vi "MainCodeSimple.vi"() -> ()   [LabVIEW 2023]
uses:
  <extravilib>/ChannelInstances/Tag-bool/Read With Abort.vi
  <extravilib>/ChannelInstances/Tag-bool/Write With Abort.vi
  <vilib>/Instr/_visa.llb/VISA Configure Serial Port (Instr).vi
  <extravilib>/ChannelInstances/Tag-bool/Instantiate.vi
  <extravilib>/ChannelInstances/Tag-bool/EndpointRead.vi
  <vilib>/Utility/file.llb/Write Delimited Spreadsheet (DBL).vi
  <extravilib>/ChannelInstances/Tag-bool/Endpoint.vi
  <extravilib>/ChannelInstances/Tag-bool.lvlib
panel:
  in  "Target temp":dbl format="%#_13g"
  in  "Massflow in, see table for ref (mV)":dbl
  in  "Opening, ouptut down (adsorption) (deg)":dbl
  in  "Opening, ouptut up (desorption) (deg)":dbl
  in  "Opening, input (deg)":dbl
  out "Temp PID":dbl(slide) scale=0.0..100.0
  in  "VISA PID":refnum<visa-resource-name>="COM6"
  out "Mode ON/OFF":bool
  out "Mode PID":bool
  in  "Switch Mode":bool
  in  "DC Pulse (ON/OFF)":bool
  in  "Sampling time (ms)":dbl format="%#_13g"
  out "Thermometer 1":dbl(slide) scale=0.0..100.0
  in  "Path":path
  in  "Save data":bool
  in  "Input massflow":dbl format="%#_13g"
  in  "C_CO2":dbl format="%#_13g"
  in  "Temp_e_3":dbl format="%#_13g"
  in  "Temp_e_2":dbl format="%#_13g"
  in  "Temp_e_1":dbl format="%#_13g"
  in  "Temp_m_3":dbl format="%#_13g"
  in  "Temp_m_2":dbl format="%#_13g"
  in  "Temp_m_1":dbl format="%#_13g"
  in  "DAC_2_1":dbl format="%#_13g"
  in  "DAC_2_0":dbl format="%#_13g"
  in  "DAC_1_1":dbl format="%#_13g"
  in  "DAC_1_0":dbl format="%#_13g"
  out "Thermometer 2":dbl(slide) scale=0.0..100.0
  out "error out 3":errorcluster
  in  "VISA Arduino":refnum<visa-resource-name>
  in  "STOP PROGRAM":bool
  # "CONTROL PANEL"
  # "Process"
  # "Serial"
  # "For the moment, mass flows under 100m^3/h are not supported"
  # "For adsorption (90°) and desorption (20°):\n-Adsorption -> 1000mV 208m^3/h\n                            1500mV 307m^3/h\n                            2000mV 406m^3/h\n                            2500mV 505m^3/h\n                            3000mV 604m^3/h\n-Desorption -> 3000mV 200m^3/h \n                           2500mV 180m^3/h \n                           2000mV 130m^3/h \n                           1500mV 100m^3/h"
  # "Careful that PID arduino are not communicating on same port"
  # "MONITORING"
  # "Data save"
  # "CURRENT ACTUATOR VALUES"
  # "PID temperature monitoring"
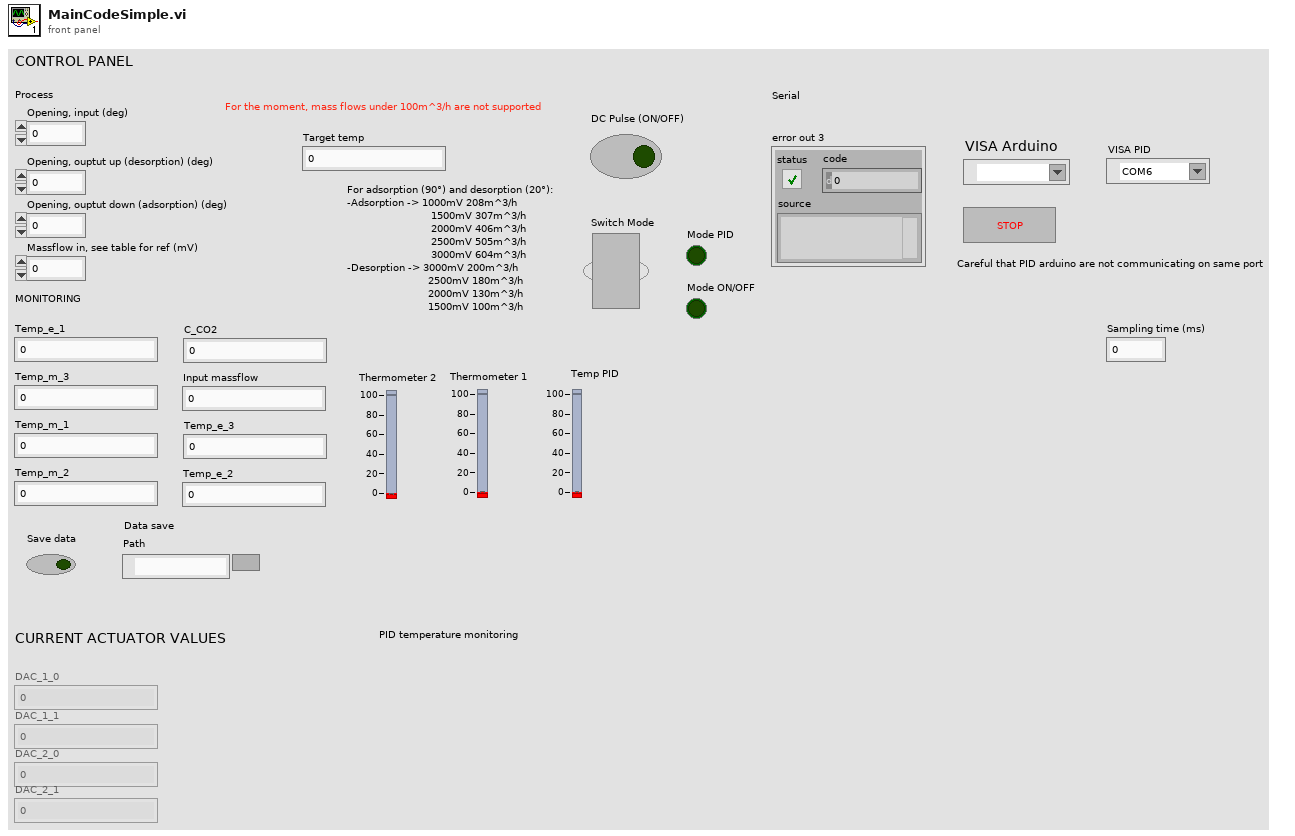
[diagram p1: front panel]
types:
  T1 = typedef "Tag-bool.lvlib/))Channel.ctl" = refnum<queue>
  T2 = cluster{"Temp_m_1":dbl, "Temp_m_2":dbl, "Temp_m_3":dbl, "Temp_e_1":dbl, "Temp_e_2":dbl, "Temp_e_3":dbl, "C_CO2":dbl, "Input massflow":dbl}
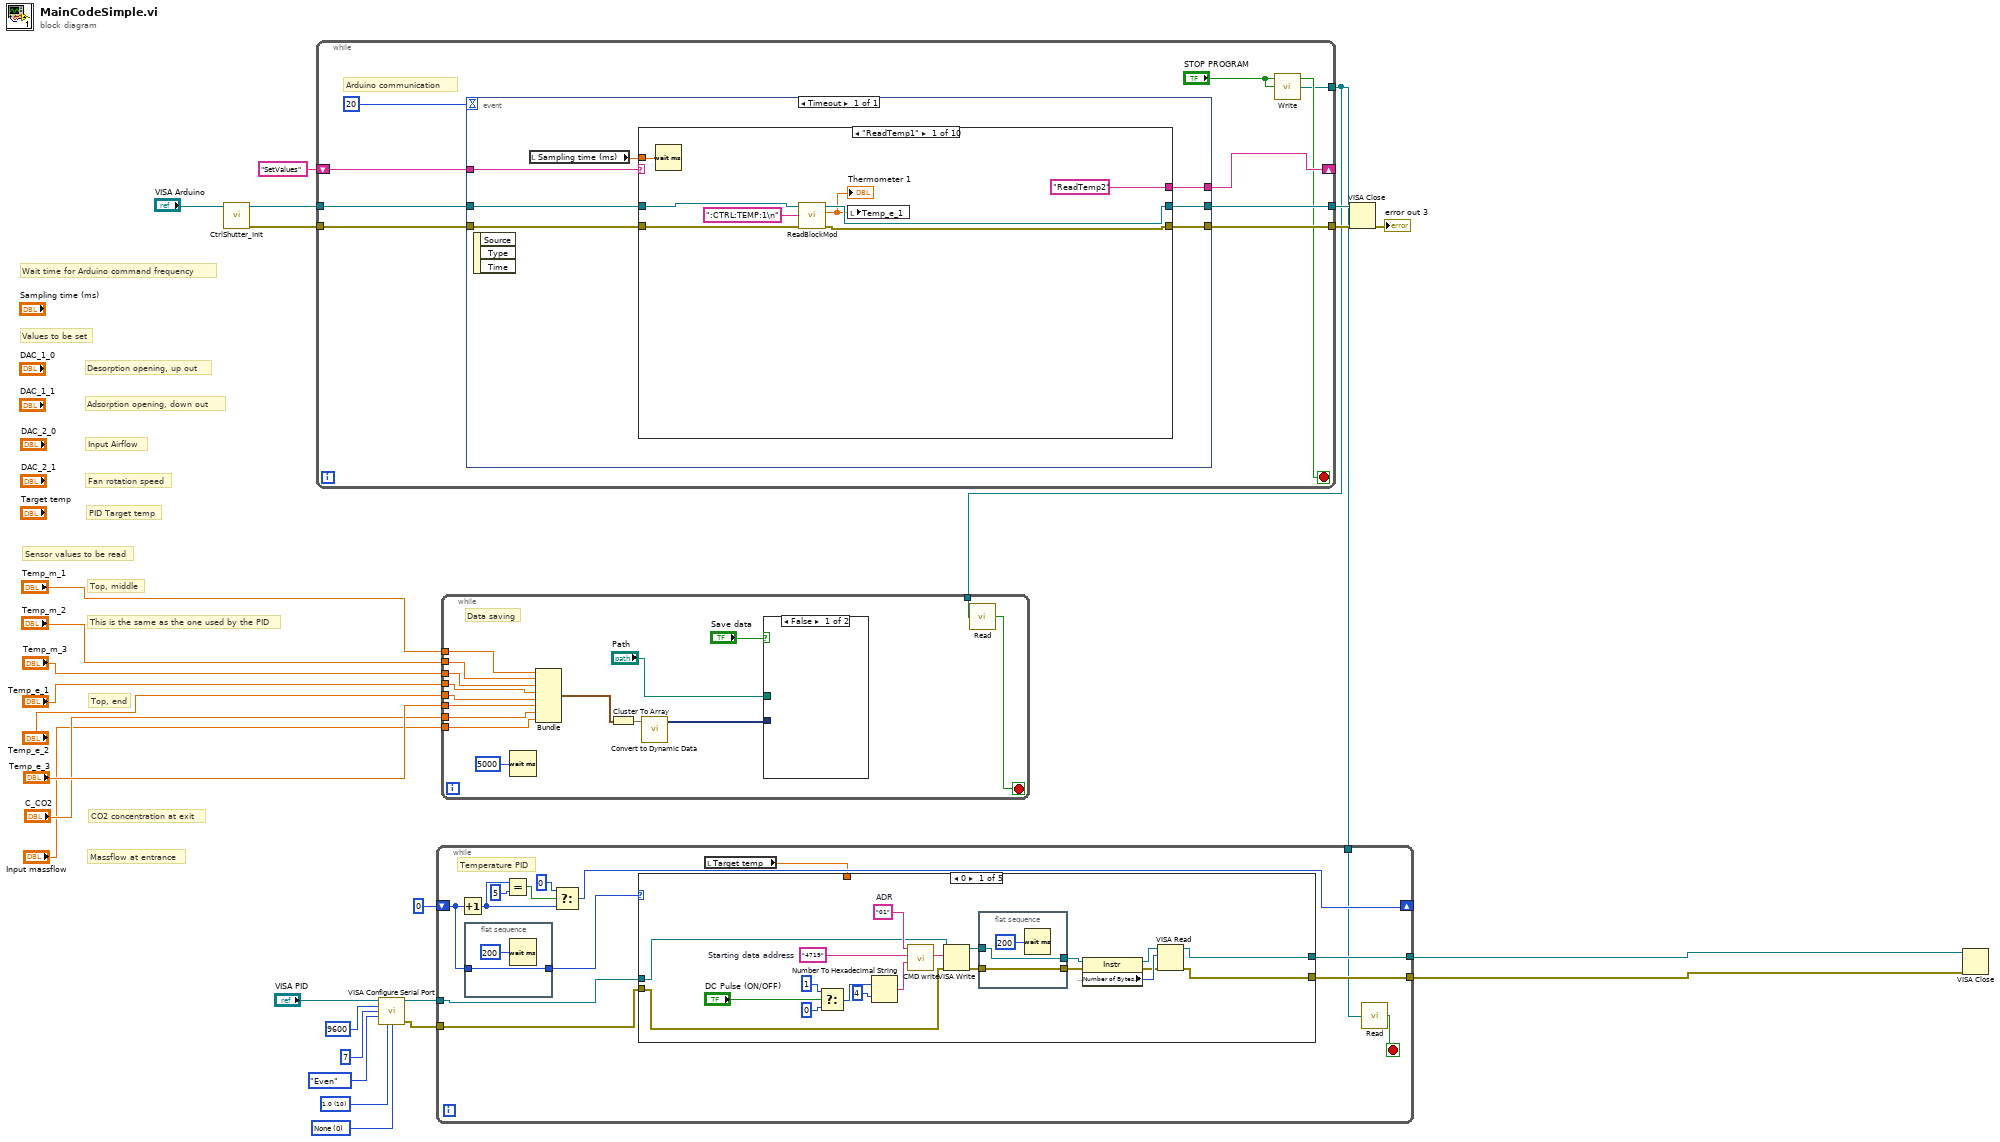
[diagram p0: block diagram]
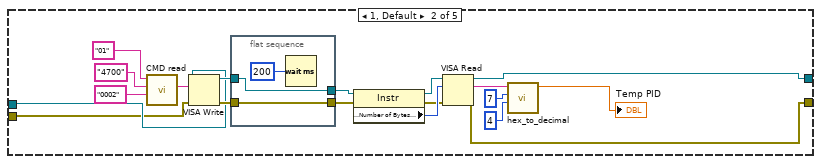
[diagram p2: hidden frame]
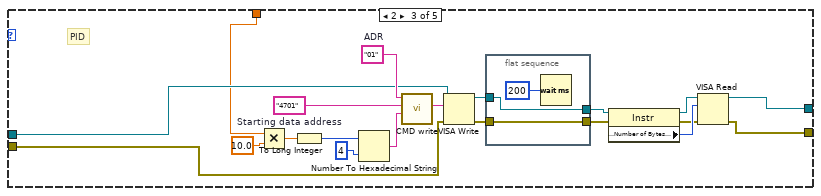
[diagram p3: hidden frame]
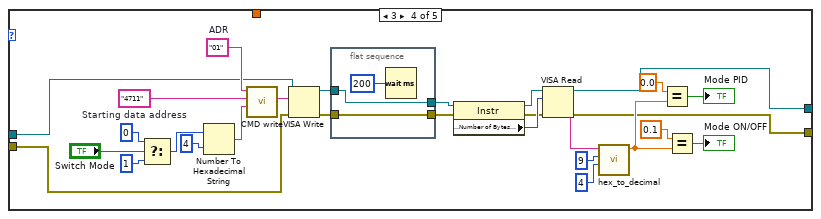
[diagram p4: hidden frame]
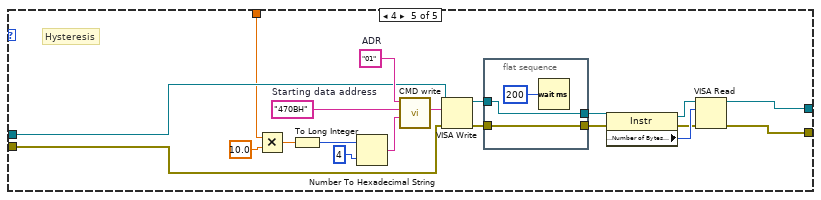
[diagram p5: hidden frame]
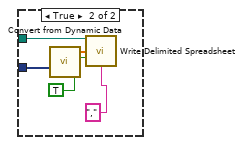
[diagram p6: hidden frame]
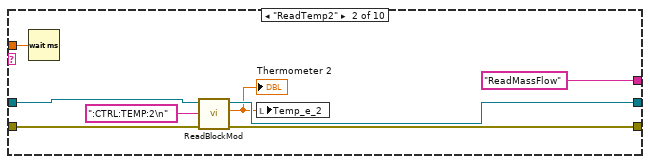
[diagram p7: hidden frame]
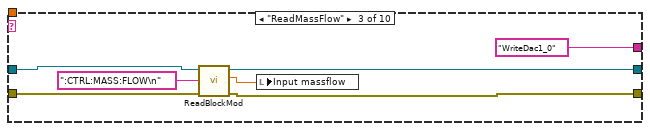
[diagram p8: hidden frame]
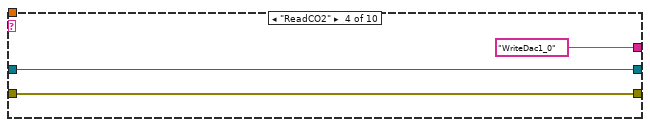
[diagram p9: hidden frame]
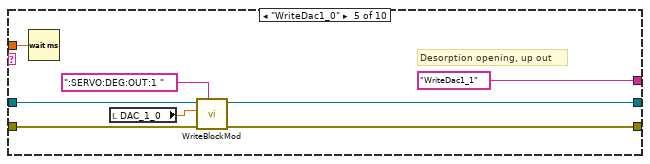
[diagram p10: hidden frame]
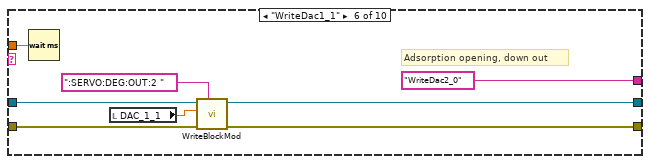
[diagram p11: hidden frame]
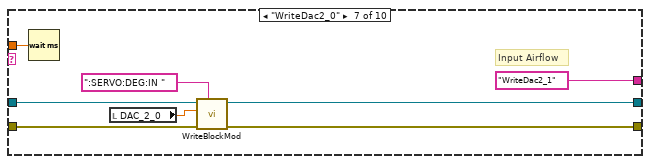
[diagram p12: hidden frame]
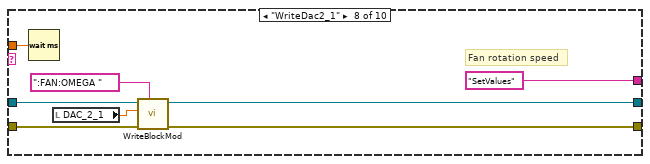
[diagram p13: hidden frame]
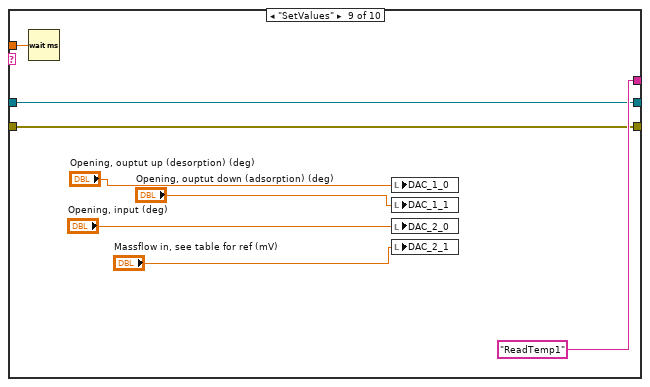
[diagram p14: hidden frame]
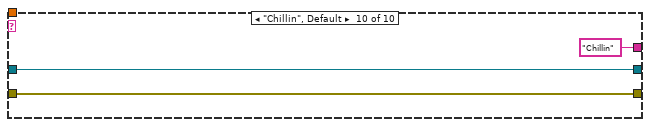
[diagram p15: hidden frame]
diagram:
  w7 = u16 0 items=["None"=0, "XON/XOFF"=1, "RTS/CTS"=2, "DTR/DSR"=4] ("flow control (0:none)")
  w8 = u16 10 items=["1.0"=10, "1.5"=15, "2.0"=20] ("stop bits (10: 1 bit)")
  # "PID Target temp"
  # "Wait time for Arduino command frequency"
  # "Massflow at entrance"
  # "CO2 concentration at exit"
  # "Top, end"
  # "This is the same as the one used by the PID"
  # "Top, middle"
  # "Sensor values to be read"
  # "Fan rotation speed"
  # "Input Airflow"
  # "Adsorption opening, down out"
  # "Desorption opening, up out"
  # "Values to be set"
  n1 = call "CtrlShutter_Init.vi"("VISA Refnum in"="VISA Arduino") -> ("error out"=w24:errorcluster, "VISA Refnum out"=w25:refnum<visa-resource-name>)  [unwired: 8 in, 1 out]
  n2 = while {
    tunnel: w25 -> [w35]
    tunnel: w24 -> [w34]
    tunnel: [w33] -> w22
    tunnel: [w32] -> w21
    shift-right: [w30] -> _
    shift-left: "SetValues" ("f") -> [w31]
    tunnel: [w28] -> w1
    stop <- "STOP PROGRAM" stop-if-true
    # "Arduino communication"
    n3 = event shown="[0] Timeout" {
      selector: _ -> [_]
      dyn-events: _ -> [_]
      timeout: 20 -> [_]
      tunnel: [w39] -> w30
      tunnel: w35 -> [w43]
      tunnel: w34 -> [w42]
      tunnel: [w41] -> w33
      tunnel: [w40] -> w32
      tunnel: w31 -> [w38]
      event Timeout {
        n4 = event-data() -> ()  [unwired: 1 in, 3 out]
        n5 = local read "Sampling time (ms)"() -> (w37:dbl)
        n6 = case shown="\"ReadTemp1\"" w38 {
          tunnel: w43 -> [w50 w55 w64 w69 w75 w84 w92 w100 w106 w110]
          tunnel: w42 -> [w49 w56 w60 w68 w71 w83 w91 w99 w107 w111]
          tunnel: [w48 w53 w62 w68 w72 w80 w88 w96 w107 w111] -> w41
          tunnel: [w47 w54 w63 w69 w73 w81 w89 w97 w106 w110] -> w40
          tunnel: ["ReadTemp2" "ReadMassFlow" "WriteDac1_0" "WriteDac1_0" "WriteDac1_1" "WriteDac2_0" "WriteDac2_1" "SetValues" "ReadTemp1" "Chillin"] -> w39
          tunnel: w37 -> [w45 w58 _ _ w76 w78 w86 w94 w109 _]
          frame "ReadTemp1" {
            n7 = Wait (ms)(milliseconds to wait=w45) -> ()  [unwired: 1 out]
            n8 = call "ReadBlockMod.vi"("VISA Refnum in"=w50, "Command"=":CTRL:TEMP:1\n", "error in (no error)"=w49) -> ("VISA Refnum out"=w47:refnum<visa-resource-name>, "Read value"=w44:dbl, "error out"=w48:errorcluster)  [unwired: 5 in]
            "Thermometer 1" <- w44
            n9 = local write "Temp_e_1"(w44) -> ()
          }
          frame "ReadTemp2" {
            n10 = Wait (ms)(milliseconds to wait=w58) -> ()  [unwired: 1 out]
            n11 = call "ReadBlockMod.vi"("VISA Refnum in"=w55, "Command"=":CTRL:TEMP:2\n", "error in (no error)"=w56) -> ("VISA Refnum out"=w54:refnum<visa-resource-name>, "Read value"=w52:dbl, "error out"=w53:errorcluster)  [unwired: 5 in]
            "Thermometer 2" <- w52
            n12 = local write "Temp_e_2"(w52) -> ()
          }
          frame "ReadMassFlow" {
            n13 = call "ReadBlockMod.vi"("VISA Refnum in"=w64, "Command"=":CTRL:MASS:FLOW\n", "error in (no error)"=w60) -> ("VISA Refnum out"=w63:refnum<visa-resource-name>, "Read value"=w61:dbl, "error out"=w62:errorcluster)  [unwired: 5 in]
            n14 = local write "Input massflow"(w61) -> ()
          }
          frame "ReadCO2" {
          }
          frame "WriteDac1_0" {
            # "Desorption opening, up out"
            n15 = Wait (ms)(milliseconds to wait=w76) -> ()  [unwired: 1 out]
            n16 = local read "DAC_1_0"() -> (w70:dbl)
            n17 = call "WriteBlockMod.vi"("VISA Refnum in"=w75, "Voltage"=w70, "error in (no error)"=w71, "Command"=":SERVO:DEG:OUT:1 ") -> ("VISA Refnum out"=w73:refnum<visa-resource-name>, "error out"=w72:errorcluster)  [unwired: 4 in, 1 out]
          }
          frame "WriteDac1_1" {
            # "Adsorption opening, down out"
            n18 = Wait (ms)(milliseconds to wait=w78) -> ()  [unwired: 1 out]
            n19 = local read "DAC_1_1"() -> (w82:dbl)
            n20 = call "WriteBlockMod.vi"("VISA Refnum in"=w84, "Voltage"=w82, "error in (no error)"=w83, "Command"=":SERVO:DEG:OUT:2 ") -> ("VISA Refnum out"=w81:refnum<visa-resource-name>, "error out"=w80:errorcluster)  [unwired: 4 in, 1 out]
          }
          frame "WriteDac2_0" {
            # "Input Airflow"
            n21 = Wait (ms)(milliseconds to wait=w86) -> ()  [unwired: 1 out]
            n22 = local read "DAC_2_0"() -> (w90:dbl)
            n23 = call "WriteBlockMod.vi"("VISA Refnum in"=w92, "Voltage"=w90, "error in (no error)"=w91, "Command"=":SERVO:DEG:IN ") -> ("VISA Refnum out"=w89:refnum<visa-resource-name>, "error out"=w88:errorcluster)  [unwired: 4 in, 1 out]
          }
          frame "WriteDac2_1" {
            # "Fan rotation speed"
            n24 = Wait (ms)(milliseconds to wait=w94) -> ()  [unwired: 1 out]
            n25 = local read "DAC_2_1"() -> (w98:dbl)
            n26 = call "WriteBlockMod.vi"("VISA Refnum in"=w100, "Voltage"=w98, "error in (no error)"=w99, "Command"=":FAN:OMEGA ") -> ("VISA Refnum out"=w97:refnum<visa-resource-name>, "error out"=w96:errorcluster)  [unwired: 4 in, 1 out]
          }
          frame "SetValues" {
            n27 = Wait (ms)(milliseconds to wait=w109) -> ()  [unwired: 1 out]
            n28 = local write "DAC_1_0"("Opening, ouptut up (desorption) (deg)") -> ()
            n29 = local write "DAC_1_1"("Opening, ouptut down (adsorption) (deg)") -> ()
            n30 = local write "DAC_2_0"("Opening, input (deg)") -> ()
            n31 = local write "DAC_2_1"("Massflow in, see table for ref (mV)") -> ()
          }
          frame "Chillin", Default {
          }
        }
      }
    }
    n32 = call <extravilib>:"Write.vi"("element"="STOP PROGRAM") -> ("channel"=w28:T1)  [unwired: 1 out]
  }
  n33 = call-poly "VISA Configure Serial Port"("VISA resource name"="VISA PID", "baud rate (9600)"=u32 9600, "data bits (8)"=u16 7, "parity (0:none)"=enum16{"None", "Odd", "Even", "Mark", "Space"}."Even", "stop bits (10: 1 bit)"=w8, "flow control (0:none)"=w7) -> ("VISA resource name out"=w6:refnum<visa-resource-name>, "error out"=w5:errorcluster)  [unwired: 2 in, 6 out]
  n34 = while {
    tunnel: w6 -> [w121]
    tunnel: w5 -> [w120]
    shift-right: [w118] -> _
    shift-left: 0 -> [w119]
    tunnel: [w117] -> w3
    tunnel: [w116] -> w2
    tunnel: w1 -> [w114]
    stop <- w115 stop-if-true
    # "Temperature PID"
    n35 = Increment(x=w119) -> (x+1=w124:i32)
    n36 = flat-sequence {
      tunnel: w119 -> [w127]
      tunnel: [w127] -> w122
      frame #0 {
        n37 = Wait (ms)(milliseconds to wait=u32 200 ("attente (ms)")) -> ()  [unwired: 1 out]
      }
    }
    n38 = Equal?(x=w124, y=5) -> (x = y?=w125:bool)
    n39 = Select(t=0, s=w125, f=w124) -> (s? t:f=w118:i32)
    n40 = local read "Target temp"() -> (w113:dbl)
    n41 = case shown="0" w122 {
      tunnel: w121 -> [w132 w156 w178 w209 w232]
      tunnel: w120 -> [w131 w155 w177 w208 w231]
      tunnel: [w130 w154 w176 w198 w230] -> w117
      tunnel: [w129 w153 w175 w197 w229] -> w116
      tunnel: w113 -> [_ _ w174 _ w228]
      frame 0 {
        w141 = "01"  # ADR
        w140 = "4719"  # Starting data address
        n42 = Select(t=1, s="DC Pulse (ON/OFF)", f=0) -> (s? t:f=w135:i32)
        n43 = Number To Hexadecimal String(1:i16 4 ("largeur (-)"), 2:w135) -> (0:w133:string)
        n44 = call "CMD write.vi"("Data Content"=w133, "Starting data address"=w140, "ADR"=w141) -> ("Chaîne en sortie"=w139:string)  [unwired: 6 in]
        n45 = VISA Write(VISA resource name=w132, write buffer=w139, error in (no error)=w131) -> (VISA resource name out=w145:refnum<visa-resource-name>, error out=w142:errorcluster)  [unwired: 1 out]
        n46 = flat-sequence {
          tunnel: w145 -> [w150]
          tunnel: [w150] -> w144
          tunnel: [w149] -> w143
          tunnel: w142 -> [w149]
          frame #0 {
            n47 = Wait (ms)(milliseconds to wait=u32 200 ("attente (ms)")) -> ()  [unwired: 1 out]
          }
        }
        n48 = property class="Instr"(reference=w144, error in=w143) -> (reference out=w148:refnum<visa-resource-name>, error out=w146:errorcluster, "Serial Settings:Number of Bytes at Serial Port"=w147:u32)
        n49 = VISA Read(VISA resource name=w148, byte count=w147, error in (no error)=w146) -> (VISA resource name out=w130:refnum<visa-resource-name>, error out=w129:errorcluster)  [unwired: 2 out]
      }
      frame 1, Default {
        n50 = call "CMD read.vi"("Data Content"="0002", "Starting data address"="4700", "ADR"="01") -> ("Chaîne en sortie"=w158:string)  [unwired: 6 in]
        n51 = VISA Write(VISA resource name=w156, write buffer=w158, error in (no error)=w155) -> (VISA resource name out=w167:refnum<visa-resource-name>, error out=w164:errorcluster)  [unwired: 1 out]
        n52 = flat-sequence {
          tunnel: w167 -> [w172]
          tunnel: [w172] -> w166
          tunnel: [w171] -> w165
          tunnel: w164 -> [w171]
          frame #0 {
            n53 = Wait (ms)(milliseconds to wait=u32 200 ("attente (ms)")) -> ()  [unwired: 1 out]
          }
        }
        n54 = property class="Instr"(reference=w166, error in=w165) -> (reference out=w170:refnum<visa-resource-name>, error out=w168:errorcluster, "Serial Settings:Number of Bytes at Serial Port"=w169:u32)
        n55 = VISA Read(VISA resource name=w170, byte count=w169, error in (no error)=w168) -> (VISA resource name out=w154:refnum<visa-resource-name>, read buffer=w157:string, error out=w153:errorcluster)  [unwired: 1 out]
        n56 = call "hex_to_decimal.vi"("length (rest)"=4, "offset (0)"=7, "read buffer"=w157) -> ("Numeric"=→"Temp PID":dbl)  [unwired: 8 in]
      }
      frame 2 {
        w182 = "01"  # ADR
        w180 = "4701"  # Starting data address
        # "PID"
        n57 = Multiply(x=w174, y=10.0) -> (x*y=w190:dbl)
        n58 = To Long Integer(number=w190) -> (32bit integer=w193:i32)
        n59 = Number To Hexadecimal String(1:i16 4 ("largeur (-)"), 2:w193) -> (0:w181:string)
        n60 = call "CMD write.vi"("Data Content"=w181, "Starting data address"=w180, "ADR"=w182) -> ("Chaîne en sortie"=w179:string)  [unwired: 6 in]
        n61 = VISA Write(VISA resource name=w178, write buffer=w179, error in (no error)=w177) -> (VISA resource name out=w186:refnum<visa-resource-name>, error out=w183:errorcluster)  [unwired: 1 out]
        n62 = flat-sequence {
          tunnel: w186 -> [w195]
          tunnel: [w195] -> w185
          tunnel: [w194] -> w184
          tunnel: w183 -> [w194]
          frame #0 {
            n63 = Wait (ms)(milliseconds to wait=u32 200 ("attente (ms)")) -> ()  [unwired: 1 out]
          }
        }
        n64 = property class="Instr"(reference=w185, error in=w184) -> (reference out=w189:refnum<visa-resource-name>, error out=w187:errorcluster, "Serial Settings:Number of Bytes at Serial Port"=w188:u32)
        n65 = VISA Read(VISA resource name=w189, byte count=w188, error in (no error)=w187) -> (VISA resource name out=w176:refnum<visa-resource-name>, error out=w175:errorcluster)  [unwired: 2 out]
      }
      frame 3 {
        w217 = "01"  # ADR
        w216 = "4711"  # Starting data address
        n66 = Select(t=0, s="Switch Mode", f=1) -> (s? t:f=w212:i32)
        n67 = Number To Hexadecimal String(1:i16 4 ("largeur (-)"), 2:w212) -> (0:w210:string)
        n68 = call "CMD write.vi"("Data Content"=w210, "Starting data address"=w216, "ADR"=w217) -> ("Chaîne en sortie"=w215:string)  [unwired: 6 in]
        n69 = VISA Write(VISA resource name=w209, write buffer=w215, error in (no error)=w208) -> (VISA resource name out=w221:refnum<visa-resource-name>, error out=w218:errorcluster)  [unwired: 1 out]
        n70 = flat-sequence {
          tunnel: w221 -> [w226]
          tunnel: [w226] -> w220
          tunnel: [w225] -> w219
          tunnel: w218 -> [w225]
          frame #0 {
            n71 = Wait (ms)(milliseconds to wait=u32 200 ("attente (ms)")) -> ()  [unwired: 1 out]
          }
        }
        n72 = property class="Instr"(reference=w220, error in=w219) -> (reference out=w224:refnum<visa-resource-name>, error out=w222:errorcluster, "Serial Settings:Number of Bytes at Serial Port"=w223:u32)
        n73 = VISA Read(VISA resource name=w224, byte count=w223, error in (no error)=w222) -> (VISA resource name out=w198:refnum<visa-resource-name>, read buffer=w205:string, error out=w197:errorcluster)  [unwired: 1 out]
        n74 = call "hex_to_decimal.vi"("length (rest)"=4, "offset (0)"=9, "read buffer"=w205) -> ("Numeric"=w203:dbl)  [unwired: 8 in]
        n75 = Equal?(x=0.0, y=w203) -> (x = y?=→"Mode PID":bool)
        n76 = Equal?(x=0.1, y=w203) -> (x = y?=→"Mode ON/OFF":bool)
      }
      frame 4 {
        w236 = "01"  # ADR
        w234 = "470BH"  # Starting data address
        # "Hysteresis"
        n77 = Multiply(x=w228, y=10.0) -> (x*y=w244:dbl)
        n78 = To Long Integer(number=w244) -> (32bit integer=w247:i32)
        n79 = Number To Hexadecimal String(1:i16 4 ("largeur (-)"), 2:w247) -> (0:w235:string)
        n80 = call "CMD write.vi"("Data Content"=w235, "Starting data address"=w234, "ADR"=w236) -> ("Chaîne en sortie"=w233:string)  [unwired: 6 in]
        n81 = VISA Write(VISA resource name=w232, write buffer=w233, error in (no error)=w231) -> (VISA resource name out=w240:refnum<visa-resource-name>, error out=w237:errorcluster)  [unwired: 1 out]
        n82 = flat-sequence {
          tunnel: w240 -> [w249]
          tunnel: [w249] -> w239
          tunnel: [w248] -> w238
          tunnel: w237 -> [w248]
          frame #0 {
            n83 = Wait (ms)(milliseconds to wait=u32 200 ("attente (ms)")) -> ()  [unwired: 1 out]
          }
        }
        n84 = property class="Instr"(reference=w239, error in=w238) -> (reference out=w243:refnum<visa-resource-name>, error out=w241:errorcluster, "Serial Settings:Number of Bytes at Serial Port"=w242:u32)
        n85 = VISA Read(VISA resource name=w243, byte count=w242, error in (no error)=w241) -> (VISA resource name out=w230:refnum<visa-resource-name>, error out=w229:errorcluster)  [unwired: 2 out]
      }
    }
    n86 = call <extravilib>:"Read.vi"("channel"=w114) -> ("element"=w115:bool)  [unwired: 1 in, 1 out]
  }
  n87 = while {
    tunnel: "Temp_m_1" -> [w264]
    tunnel: "Temp_m_2" -> [w263]
    tunnel: "Temp_m_3" -> [w259]
    tunnel: "Temp_e_1" -> [w258]
    tunnel: "Temp_e_2" -> [w257]
    tunnel: "Temp_e_3" -> [w256]
    tunnel: "C_CO2" -> [w255]
    tunnel: "Input massflow" -> [w254]
    tunnel: w1 -> [w260]
    stop <- w266 stop-if-true
    # "Data saving"
    n88 = Wait (ms)(milliseconds to wait=u32 5000) -> ()  [unwired: 1 out]
    n89 = Bundle("Temp_m_1"=w264, "Temp_m_2"=w263, "Temp_m_3"=w259, "Temp_e_1"=w258, "Temp_e_2"=w257, "Temp_e_3"=w256, "C_CO2"=w255, "Input massflow"=w254) -> (w253:T2)  [unwired: 1 in]
    n90 = Cluster To Array(cluster=w253) -> (array=w261:dbl[])
    n91 = call "Convert to Dynamic Data"("Array"=w261) -> ("Dynamic Data Type"=w252:dynamicdata)  [unwired: 3 in]
    n92 = case shown="False" "Save data" {
      tunnel: w252 -> [_ w271]
      tunnel: "Path" -> [_ w269]
      frame False {
      }
      frame True {
        n93 = call "Convert from Dynamic Data"("Dynamic Data Type"=w271) -> ("Array"=w270:dbl[])  [unwired: 3 in]
        n94 = call-poly <vilib>:"Write Delimited Spreadsheet.vi"("file path (dialog if empty)"=w269, "1D data"=w270, "append to file? (new file:F)"=TRUE, "delimiter (\\t)"=",") -> ()  [unwired: 10 in, 2 out]
      }
    }
    n95 = call <extravilib>:"Read.vi"("channel"=w260) -> ("element"=w266:bool)  [unwired: 1 in, 1 out]
  }
  n96 = VISA Close(VISA resource name=w21, error in (no error)=w22) -> (error out=→"error out 3":errorcluster)
  n97 = VISA Close(VISA resource name=w3, error in (no error)=w2) -> ()  [unwired: 1 out]
